vi "4bar setpoint and immediate.vi"(4 "Cargo Ship for Cargo":dbl, 6 "Operator X Button":bool, 7 "Hatch Setpoint":dbl, 8 "Operator Y Button":bool, 9 "Operator B Button":bool, 10 "Operator A Button":bool, 11 "Operator Right Joystick Y in":dbl) -> (3 "Output":cluster{"Control Mode":T1, "Output":dbl} {"Control Mode" items=["PercentOutput"=0, "Position"=1, "Velocity"=2, "Current"=3, "Follower"=5, "MotionProfile"=6, "MotionMagic"=7, "MotionProfileArc"=10, "Disabled"=15]})   [LabVIEW 2018]
uses:
  <vilib>/Rock Robotics/WPI/ThirdParty/Phoenix-LabVIEW/Motor Controller/Controls/CTRE_Phoenix_MotorControl_ControlMode.ctl
  4barCommands.ctl
  Infrastructure/Constants.vi
  Robot Global Data.vi
  <vilib>/Rock Robotics/Network Tables/NT Write Number.vi
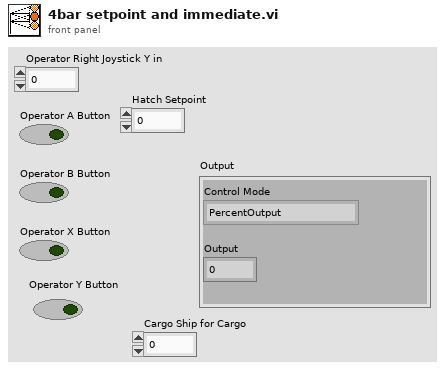
[diagram p1: front panel]
types:
  T1 = typedef "CTRE_Phoenix_MotorControl_ControlMode.ctl" = u16
  T2 = typedef "4barCommands.ctl" = enum16{"Immediate", "Hold", "Setpoint"}
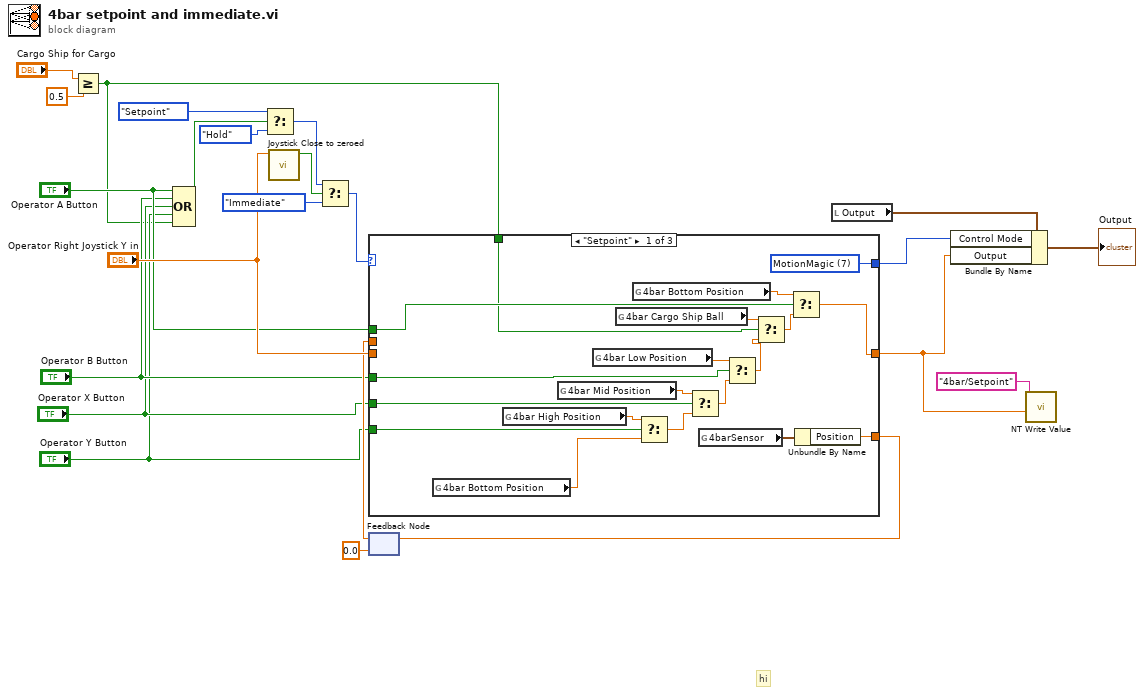
[diagram p0: block diagram]
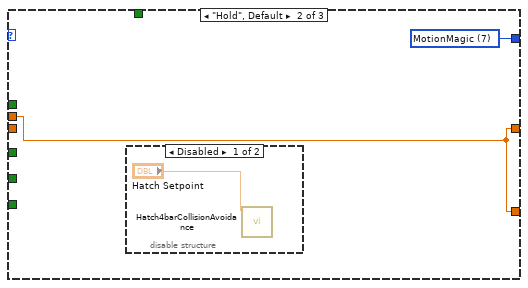
[diagram p2: hidden frame]
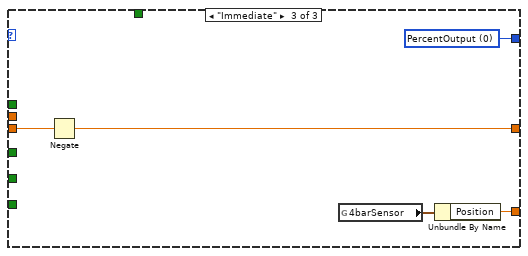
[diagram p4: hidden frame]
diagram:
  # "hi"
  n1 = Greater Or Equal?(x="Cargo Ship for Cargo", y=0.5 ("Position")) -> (x >= y?=w1:bool)
  n2 = Compound Arithmetic op=OR("Operator A Button", "Operator B Button", "Operator X Button", "Operator Y Button", w1) -> (w8:bool)
  n3 = Select(t=4barCommands."Setpoint", s=w8, f=4barCommands."Hold" ("t")) -> (s? t:f=w17:T2)
  n4 = call "Joystick Close to zeroed.vi"("Joystick"="Operator Right Joystick Y in") -> ("=0?"=w15:bool)  [unwired: 10 in]
  n5 = Select(t=w17, s=w15, f=4barCommands."Immediate") -> (s? t:f=w22:T2)
  n6 = feedback #1(0.0 ("Position")) -> (w18:dbl)
  n7 = case shown="\"Setpoint\"" w22 {
    tunnel: "Operator X Button" -> [w39 _ _]
    tunnel: "Operator B Button" -> [w25 _ _]
    tunnel: "Operator A Button" -> [w38 _ _]
    tunnel: "Operator Right Joystick Y in" -> [_ _ w49]
    tunnel: [w37 w44 w50] -> w19
    tunnel: [w24 w43 w48] -> w4
    tunnel: "Operator Y Button" -> [w35 _ _]
    tunnel: w18 -> [_ w43 _]
    tunnel: [w31 w43 w46] -> w7
    tunnel: w1 -> [w26 _ _]
    frame "Setpoint" {
      w37 = T1 7 items=["PercentOutput"=0, "Position"=1, "Velocity"=2, "Current"=3, "Follower"=5, "MotionProfile"=6, "MotionMagic"=7, "MotionProfileArc"=10, "Disabled"=15] ("Control Mode")
      n8 = global read "Constants.vi" "4bar Bottom Position"() -> (w30:dbl)
      n9 = global read "Constants.vi" "4bar High Position"() -> (w36:dbl)
      n10 = global read "Constants.vi" "4bar Mid Position"() -> (w42:dbl)
      n11 = global read "Constants.vi" "4bar Low Position"() -> (w29:dbl)
      n12 = global read "Constants.vi" "4bar Cargo Ship Ball"() -> (w41:dbl)
      n13 = global read "Constants.vi" "4bar Bottom Position"() -> (w40:dbl)
      n14 = Select(t=w36, s=w35, f=w30) -> (s? t:f=w34:dbl)
      n15 = Select(t=w42, s=w39, f=w34) -> (s? t:f=w28:dbl)
      n16 = global read "Robot Global Data.vi" "4barSensor"() -> (w32:cluster{"Position":dbl, "Velocity":dbl})
      n17 = Select(t=w29, s=w25, f=w28) -> (s? t:f=w27:dbl)
      n18 = Select(t=w41, s=w26, f=w27) -> (s? t:f=w33:dbl)
      n19 = Select(t=w40, s=w38, f=w33) -> (s? t:f=w24:dbl)
      n20 = Unbundle By Name(w32) -> ("Position"=w31:dbl)
    }
    frame "Hold", Default {
      w44 = T1 7 items=["PercentOutput"=0, "Position"=1, "Velocity"=2, "Current"=3, "Follower"=5, "MotionProfile"=6, "MotionMagic"=7, "MotionProfileArc"=10, "Disabled"=15] ("Control Mode")
      n21 = disable-structure shown="Disabled" {
        frame Disabled {
          n22 = call "Hatch4barCollisionAvoidance.vi"("Hatch Setpoint"="Hatch Setpoint") -> ()  [unwired: 10 in, 1 out]
        }
        frame Enabled {
        }
      }
    }
    frame "Immediate" {
      w50 = T1 0 items=["PercentOutput"=0, "Position"=1, "Velocity"=2, "Current"=3, "Follower"=5, "MotionProfile"=6, "MotionMagic"=7, "MotionProfileArc"=10, "Disabled"=15] ("Control Mode")
      n23 = Negate(x=w49) -> (-x=w48:dbl)
      n24 = global read "Robot Global Data.vi" "4barSensor"() -> (w47:cluster{"Position":dbl, "Velocity":dbl})
      n25 = Unbundle By Name(w47) -> ("Position"=w46:dbl)
    }
  }
  n26 = feedback-in #1(w7) -> ()
  n27 = local read "Output"() -> (w20:cluster{"Control Mode":T1, "Output":dbl})
  n28 = Bundle By Name(cluster=w20, "Control Mode"=w19, "Output"=w4) -> (→"Output":cluster{"Control Mode":T1, "Output":dbl})
  n29 = call-poly <vilib>:"NT Write Value.vi"("Numeric"=w4, "Name"="4bar/Setpoint") -> ()  [unwired: 9 in, 1 out]
